vi "Configure Frequency.vi"(8 "error in (no error)":errorcluster, 10 "Frequency [Hz]":dbl, 11 "SigGen-8665B in":refnum<class "SigGen-8665B.lvclass">) -> (0 "error out":errorcluster, 3 "SigGen-8665B out":refnum<class "SigGen-8665B.lvclass">)   [LabVIEW 2020, in "SigGen-8665B.lvclass"]
uses:
  SigGen-8665B.lvclass
  C:/Sandbox/RF Bench/Source Code/WiSpry Test Framework/Instruments/Signal Generator/Signal Generator.lvclass
  C:/Sandbox/RF Bench/Source Code/WiSpry Test Framework/Instruments/Instrument.lvclass
  Signal Generator.lvclass/Signal Generator.ctl
  Instrument.lvclass/Instrument.ctl
  Instrument.lvclass
  Signal Generator.lvclass
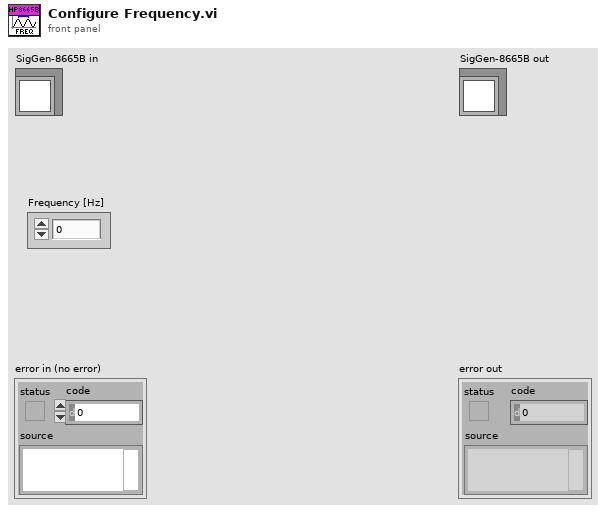
[diagram p1: front panel]
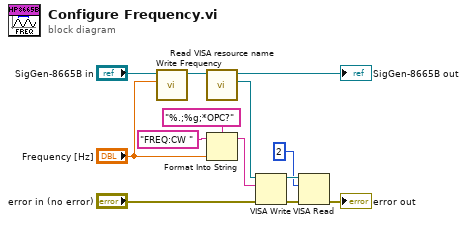
[diagram p0: block diagram]
diagram:
  n1 = call "Write Frequency.vi"("Frequency"="Frequency [Hz]", "Signal Generator in"="SigGen-8665B in") -> ("Signal Generator out"=w2:refnum<class "SigGen-8665B.lvclass">)  [unwired: 9 in]
  n2 = call "Read VISA resource name.vi"("Instrument in"=w2) -> ("VISA resource name"=w10:refnum<visa-resource-name>, "Instrument out"=→"SigGen-8665B out":refnum<class "SigGen-8665B.lvclass">)  [unwired: 9 in]
  n3 = Format Into String(format string="%.;%g;*OPC?", initial string="FREQ:CW ", "Frequency [Hz]") -> (resulting string=w8:string)  [unwired: 1 in, 1 out]
  n4 = VISA Write(VISA resource name=w10, write buffer=w8, error in (no error)="error in (no error)") -> (VISA resource name out=w6:refnum<visa-resource-name>, error out=w7:errorcluster)  [unwired: 1 out]
  n5 = VISA Read(VISA resource name=w6, byte count=u32 2, error in (no error)=w7) -> (error out=→"error out":errorcluster)  [unwired: 3 out]
